vi "DER_Control_subTest.vi"(7 "Test Result in":T2=enum."Success", 8 "error in":errorcluster, 9 "DeviceID":T1, 10 "MicrogridID":u8, 11 "Message Enqueuer in":refnum<class "Message Enqueuer.lvclass">) -> (0 "error out":errorcluster, 1 "dup DeviceID":T1, 2 "dup MicrogridID":u8, 3 "Message Enqueuer out":refnum<class "Message Enqueuer.lvclass">, 5 "Test Result out":T2=enum."Success")   [LabVIEW 2018, in "IED Test Framework.lvlib" / "IED Test.lvclass"]
doc: "This VI tests Activate and Deactive messages as part of DER_Control."
uses:
  IED Test.lvclass
  Controls/Test Result.ctl
  <vilib>/ORNL/CSEISMIC DDS/CSEISMIC DDS Base/Data Types/Controls/DeviceID.ctl
  <vilib>/ActorFramework/Message Enqueuer/Message Enqueuer.lvclass
  <vilib>/ORNL/CSEISMIC DDS/CSEISMIC DDS Base/Data Types/DER_Control.ctl
  <vilib>/ORNL/CSEISMIC DDS/CSEISMIC DDS Base/CSEISMIC DDS.lvclass/CSEISMIC DDS.ctl
  <vilib>/ORNL/CSEISMIC DDS/CSEISMIC DDS Base/Accessors/Write DDS Reference.vi
  <vilib>/ORNL/CSEISMIC DDS/CSEISMIC DDS Base/Accessors/Read DDS Reference.vi
  <vilib>/ORNL/CSEISMIC DDS/DDS Reader/DDS Reader.lvclass
  C:/Program Files (x86)/National Instruments/LabVIEW 2018/vi.lib/ORNL/CSEISMIC DDS/CSEISMIC DDS Base/CSEISMIC DDS.lvclass
  <vilib>/ORNL/CSEISMIC DDS/CSEISMIC DDS Base/Error Handler.vi
  DER Actor/DER Messages/Activate DER Msg/Activate DER Msg.lvclass
  <vilib>/ORNL/CSEISMIC DDS/CSEISMIC DDS Base/CSEISMIC DDS.lvclass
  DER Actor/DER Messages/Deactivate DER Msg/Deactivate DER Msg.lvclass
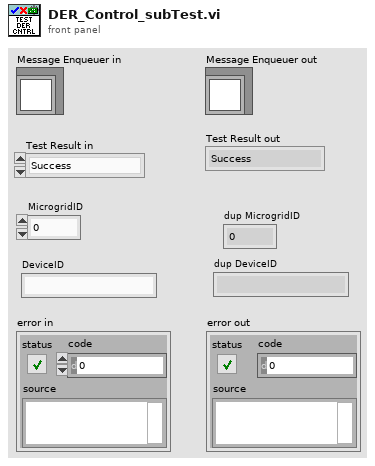
[diagram p1: front panel]
types:
  T1 = typedef "CSEISMIC DDS.lvlib/CSEISMIC DDS.lvclass/DeviceID.ctl" = string
  T2 = typedef "IED Test Framework.lvlib/IED Test.lvclass/Test Result.ctl" = enum16{"Invalid", "Success", "Failure", "Error", "Timeout"}
  T3 = typedef "CSEISMIC DDS.lvlib/CSEISMIC DDS.lvclass/DER_Control.ctl" = cluster{"DeviceID":T1, "Activate":bool, "Deactivate":bool}
  T4 = typedef "LVDDS_library.lvlib/DDS Sample Info.ctl" = cluster{"DDS_SampleStateKind":enum32{"DDS_INVALID_SAMPLE_STATE", "DDS_READ_SAMPLE_STATE", "DDS_NOT_READ_SAMPLE_STATE"}, "DDS_ViewStateKind":enum32{"DDS_INVALID_SAMPLE_STATE", "DDS_NEW_VIEW_STATE", "DDS_NOT_NEW_VIEW_STATE"}, "DDS_InstanceStateKind":enum32{"DDS_INVALID_STATE", "DDS_ALIVE_INSTANCE_STATE", "DDS_NOT_ALIVE_DISPOSED_INSTANCE_STATE", "", "DDS_NOT_ALIVE_NO_WRITERS_INSTANCE_STATE"}, "sec":i32, "nanosec":u32, "valid_data":bool}
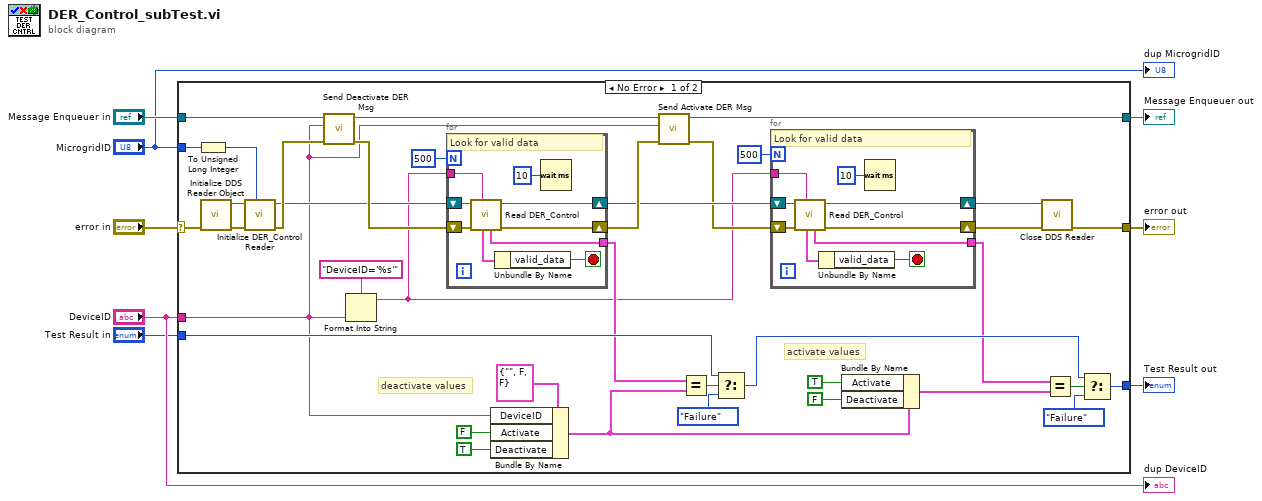
[diagram p0: block diagram]
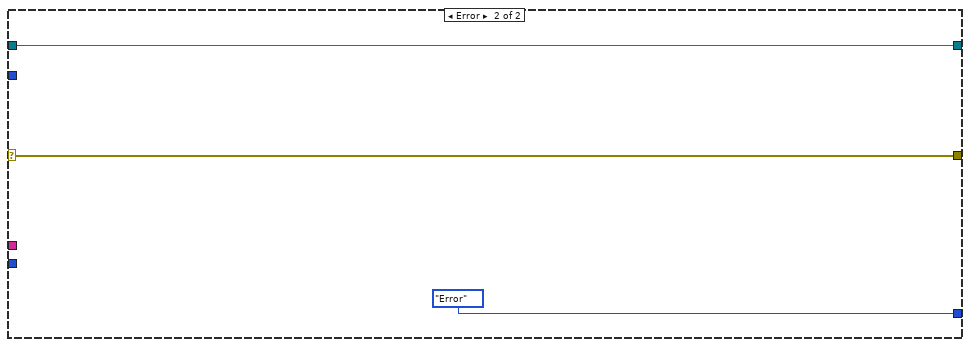
[diagram p2: hidden frame]
diagram:
  n1 = case shown="No Error" "error in" {
    selector: "error in" -> [w32 w66]
    tunnel: [w46 Test_Result."Error" ("Test Result")] -> w8
    tunnel: "DeviceID" -> [w9 _]
    tunnel: [w37 w65] -> w7
    tunnel: "MicrogridID" -> [w28 _]
    tunnel: [w24 w66] -> w6
    tunnel: "Message Enqueuer in" -> [w35 w65]
    tunnel: "Test Result in" -> [w33 _]
    frame No Error {
      # "activate values"
      # "deactivate values"
      n2 = To Unsigned Long Integer(number=w28) -> (unsigned 32bit integer=w23:u32)
      n3 = call <vilib>:"Initialize DDS Reader Object.vi"("error in"=w32) -> ("error out"=w30:errorcluster, "DDS Reader out"=w29:refnum<class "DDS Reader.lvclass">)  [unwired: 9 in]
      n4 = call <vilib>:"Initialize DER_Control Reader.vi"("MicrogridID"=w23, "error in"=w30, "DDS Reader in"=w29) -> ("error out"=w31:errorcluster, "DDS Reader out"=w26:refnum<class "DDS Reader.lvclass">)  [unwired: 7 in]
      n5 = call "Send Deactivate DER Msg.vi"("error in (no error)"=w31, "DeviceID"=w9, "Message Enqueuer in"=w35) -> ("error out"=w36:errorcluster, "Message Enqueuer out"=w34:refnum<class "Message Enqueuer.lvclass">)  [unwired: 7 in]
      n6 = Format Into String(format string="DeviceID='%s'", w9) -> (resulting string=w14:string)  [unwired: 2 in, 1 out]
      n7 = for {
        N: 500 -> [_]
        tunnel: [w61] -> w25
        shift-right: [w63] -> w27
        shift-left: w36 -> [w64]
        shift-right: [w60] -> w19
        shift-left: w26 -> [w62]
        tunnel: w14 -> [w56]
        stop <- w57 stop-if-true
        # "Look for valid data"
        n8 = call <vilib>:"Read DER_Control.vi"("Query condition"=w56, "error in"=w64, "DDS Reader in"=w62) -> ("error out"=w63:errorcluster, "DDS Reader out"=w60:refnum<class "DDS Reader.lvclass">, "data"=w61:T3, "DDS Sample Info"=w58:T4)  [unwired: 5 in]
        n9 = Unbundle By Name(w58) -> ("valid_data"=w57:bool)
        n10 = Wait (ms)(milliseconds to wait=u32 10) -> ()  [unwired: 1 out]
      }
      n11 = Bundle By Name(cluster=T3 {"DeviceID"="", "Activate"=FALSE, "Deactivate"=FALSE} ("DER_Control"), "DeviceID"=w9, "Activate"=FALSE, "Deactivate"=TRUE) -> (w11:T3)
      n12 = call "Send Activate DER Msg.vi"("error in (no error)"=w27, "DeviceID"=w9, "Message Enqueuer in"=w34) -> ("error out"=w18:errorcluster, "Message Enqueuer out"=w37:refnum<class "Message Enqueuer.lvclass">)  [unwired: 7 in]
      n13 = Equal?(x=w25, y=w11) -> (x = y?=w41:bool)
      n14 = Select(t=w33, s=w41, f=Test_Result."Failure" ("Test Result")) -> (s? t:f=w45:T2)
      n15 = for {
        N: 500 -> [_]
        tunnel: [w52] -> w17
        shift-right: [w54] -> w15
        shift-left: w18 -> [w55]
        shift-right: [w51] -> w16
        shift-left: w19 -> [w53]
        tunnel: w14 -> [w47]
        stop <- w48 stop-if-true
        # "Look for valid data"
        n16 = call <vilib>:"Read DER_Control.vi"("Query condition"=w47, "error in"=w55, "DDS Reader in"=w53) -> ("error out"=w54:errorcluster, "DDS Reader out"=w51:refnum<class "DDS Reader.lvclass">, "data"=w52:T3, "DDS Sample Info"=w49:T4)  [unwired: 5 in]
        n17 = Unbundle By Name(w49) -> ("valid_data"=w48:bool)
        n18 = Wait (ms)(milliseconds to wait=u32 10) -> ()  [unwired: 1 out]
      }
      n19 = Bundle By Name(cluster=w11, "Activate"=TRUE, "Deactivate"=FALSE) -> (w10:T3)
      n20 = call <vilib>:"Close DDS Reader.vi"("error in"=w15, "DDS Reader in"=w16) -> ("error out"=w24:errorcluster)  [unwired: 9 in]
      n21 = Equal?(x=w17, y=w10) -> (x = y?=w44:bool)
      n22 = Select(t=w45, s=w44, f=Test_Result."Failure" ("Test Result")) -> (s? t:f=w46:T2)
    }
    frame Error {
    }
  }
  "Test Result out" <- w8
  "Message Enqueuer out" <- w7
  "error out" <- w6
  "dup MicrogridID" <- "MicrogridID"
  "dup DeviceID" <- "DeviceID"
